vi "Reset Slots.vi"(8 "error in (no error)":errorcluster, 11 "Item Ref in":T1 format="%.0x") -> (0 "error out":errorcluster, 3 "Item Ref out":T1 format="%.0x")   [LabVIEW 2020, in "SEECD System Explorer.lvlib"]
uses:
  SEECD System Explorer.lvlib
  <vilib>/NI VeriStand/Custom Device API/Custom Device Item Ref.ctl
  Shared/Globals/Scan Engine GUIDs.vi
  <vilib>/NI VeriStand/Custom Device API/Custom Device API.lvlib
  Shared/SEECD Shared.lvlib
  Includes/Modules.lvlibp/RSI Module/RSI Module.lvclass
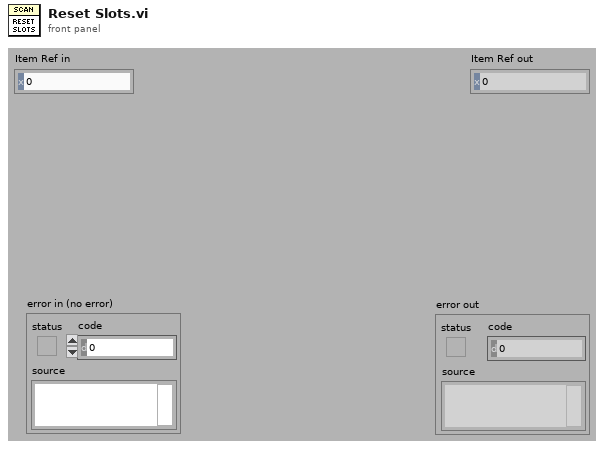
[diagram p1: front panel]
types:
  T1 = typedef "Custom Device API.lvlib/Custom Device Item Ref.ctl" = u64
  T2 = typedef "Modules.lvlibp/Custom Device API.lvlib/Custom Device Item Ref.ctl" = u64
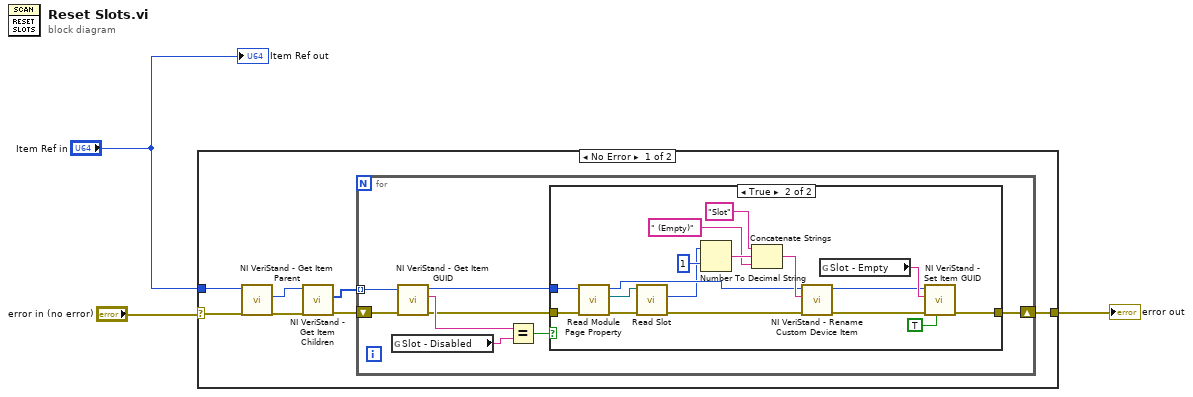
[diagram p0: block diagram]
diagram:
  n1 = case shown="No Error" "error in (no error)" {
    selector: "error in (no error)" -> [w9 w37]
    tunnel: [w4 w37] -> w2
    tunnel: "Item Ref in" -> [w10 _]
    frame No Error {
      n2 = call <vilib>:"NI VeriStand - Get Item Parent.vi"("error in (no error)"=w9, "Item Ref in"=w10) -> ("error out"=w8:errorcluster, "Parent Ref"=w7:T1)  [unwired: 6 in, 2 out]
      n3 = call <vilib>:"NI VeriStand - Get Item Children.vi"("error in (no error)"=w8, "Item Ref in"=w7) -> ("error out"=w6:errorcluster, "Child Refs"=w5:T1[])  [unwired: 6 in, 2 out]
      n4 = for {
        shift-right: [w11] -> w4
        shift-left: w6 -> [w18]
        tunnel: w5 -> [w17] mode=indexing
        n5 = global read "Scan Engine GUIDs.vi" "Slot - Disabled"() -> (w15:string)
        n6 = call <vilib>:"NI VeriStand - Get Item GUID.vi"("error in (no error)"=w18, "Item Ref in"=w17) -> ("error out"=w13:errorcluster, "GUID"=w16:string, "Item Ref out"=w12:T1)  [unwired: 7 in]
        n7 = Equal?(x=w16, y=w15) -> (x = y?=w14:bool)
        n8 = case shown="True" w14 {
          tunnel: w13 -> [w19 w28]
          tunnel: w12 -> [_ w29]
          tunnel: [w19 w34] -> w11
          frame False {
          }
          frame True {
            n9 = call "Read Module Page Property.vi"("error in (no error)"=w28, "Node Ptr In"=w29) -> ("error out"=w31:errorcluster, "RSI Module"=w30:refnum<class "RSI Module.lvclass">, "Node Ptr Out"=w22:T2)  [unwired: 7 in]
            n10 = call "Read Slot.vi"("error in (no error)"=w31, "RSI Module in"=w30) -> ("error out"=w20:errorcluster, "Slot"=w21:u32)  [unwired: 7 in, 1 out]
            n11 = Number To Decimal String(number=w21, width (-)=i16 1) -> (decimal integer string=w26:string)
            n12 = Concatenate Strings("Slot" ("string"), w26, " (Empty)" ("Section Name")) -> (w23:string)
            n13 = call <vilib>:"NI VeriStand - Rename Custom Device Item.vi"("error in (no error)"=w20, "New Name"=w23, "Item Ref in"=w22) -> ("error out"=w33:errorcluster, "Item Ref out"=w32:T1)  [unwired: 1 in, 6 out]
            n14 = global read "Scan Engine GUIDs.vi" "Slot - Empty"() -> (w35:string)
            n15 = call <vilib>:"NI VeriStand - Set Item GUID.vi"("Refresh System Explorer Tree? (F)"=TRUE, "error in (no error)"=w33, "GUID"=w35, "Item Ref in"=w32) -> ("error out"=w34:errorcluster)  [unwired: 6 in, 1 out]
          }
        }
      }
    }
    frame Error {
    }
  }
  "error out" <- w2
  "Item Ref out" <- "Item Ref in"
